vi "Qubit Count.vi"(7 "QuWire in":refnum<class "QuWire.lvclass">) -> (8 "Qubit Count":i32)   [LabVIEW 2020]
uses:
  QuSim/QuWire/QuWire.lvclass
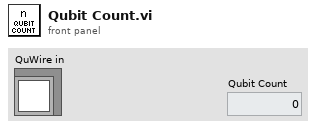
[diagram p1: front panel]
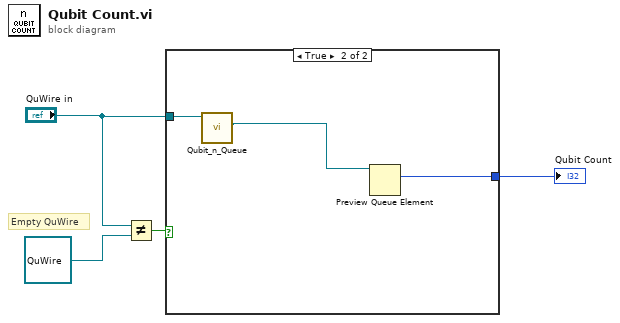
[diagram p0: block diagram]
diagram:
  # "Empty QuWire"
  n1 = Not Equal?(x="QuWire in", y=refnum<class "QuWire.lvclass"> refnum ("QuWire in")) -> (x != y?=w3:bool)
  n2 = case shown="True" w3 {
    tunnel: "QuWire in" -> [_ w7]
    tunnel: [_ w5] -> w1
    frame False {
    }
    frame True {
      n3 = call "Qubit_n_Queue.vi"("QuWire in"=w7) -> ("Qubit n"=w6:refnum<queue>)  [unwired: 8 in, 2 out]
      n4 = Preview Queue Element(queue=w6) -> (element=w5:i32)  [unwired: 2 in, 3 out]
    }
  }
  "Qubit Count" <- w1
